vi "Switch Scalar Type.vi"(8 "error in (no error)":errorcluster, 11 "Node Ptr":u64 format="%.0x") -> (0 "error out":errorcluster)   [LabVIEW 2016, in "FPGA Addon System Explorer.lvlib"]
uses:
  FPGA Addon System Explorer.lvlib
  <vilib>/NI Veristand/Custom Device API/Custom Device Channel.ctl
  <vilib>/NI Veristand/Custom Device API/Custom Device Channel Type.ctl
  Shared/Constants.vi
  <vilib>/NI Veristand/Custom Device API/Get Item Property (String).vi
  <vilib>/NI Veristand/Custom Device API/Set Item Property (String).vi
  <vilib>/NI VeriStand/Custom Device API/Custom Device API.lvlib
  Shared/FPGA Addon Shared.lvlib
  <vilib>/NI VeriStand/Custom Device Tools/Custom Device Utility Library/Custom Device Utility Library.lvlib
panel:
  in  "Tag":string
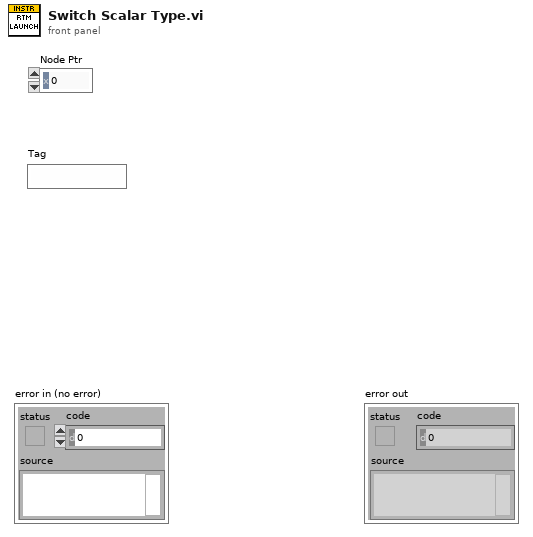
[diagram p1: front panel]
types:
  T1 = typedef "Custom Device API.lvlib/Custom Device Item Ref.ctl" = u64
  T2 = typedef "Custom Device API.lvlib/Custom Device Item Info.ctl" = cluster{"Name":string, "Is Channel":bool, "GUID":string, "Is Waveform":bool}
  T3 = typedef "Custom Device API.lvlib/Custom Device Channel.ctl" = cluster{"Type":T4, "Units":string, "Default Value":dbl, "Faultable":bool, "Scalable":bool}
  T4 = typedef "Custom Device API.lvlib/Custom Device Channel Type.ctl" = enum16{"Input", "Output"}
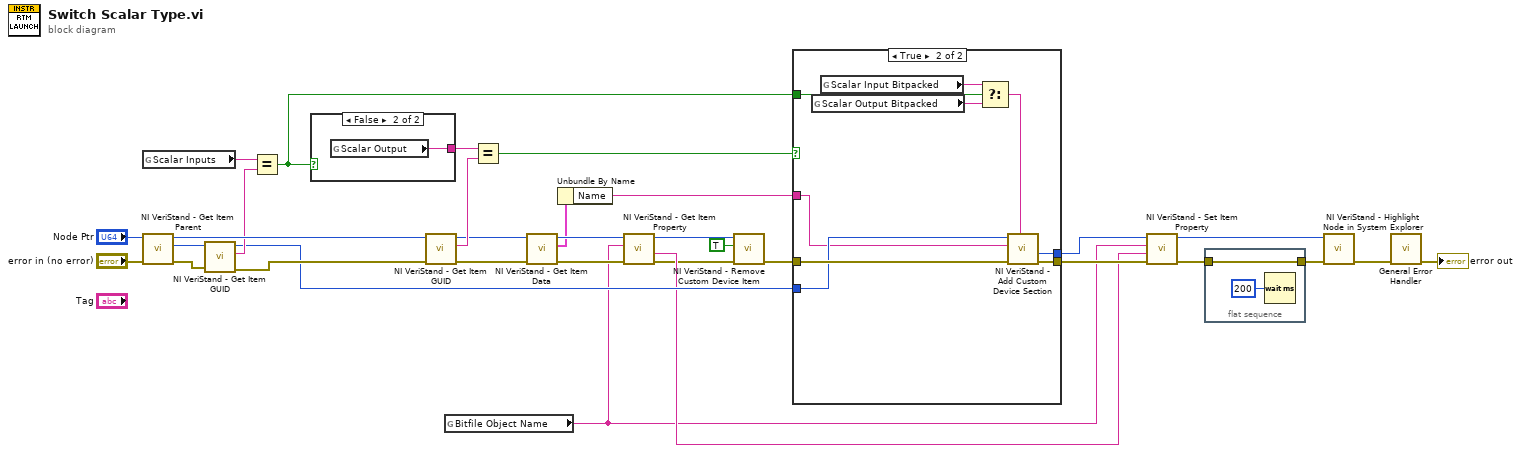
[diagram p0: block diagram]
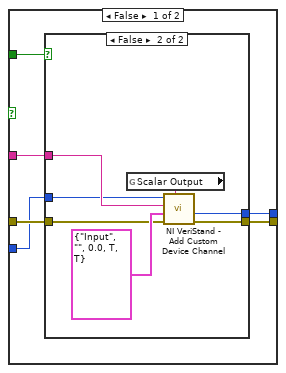
[diagram p2: hidden frame]
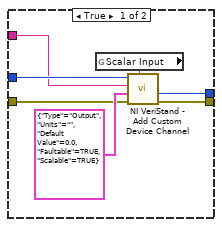
[diagram p3: hidden frame]
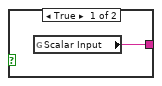
[diagram p4: hidden frame]
diagram:
  n1 = global read "Constants.vi" "Scalar Inputs"() -> (w23:string)
  n2 = call <vilib>:"NI VeriStand - Get Item Parent.vi"("error in (no error)"="error in (no error)", "Item Ref in"="Node Ptr") -> ("error out"=w25:errorcluster, "Parent Ref"=w26:T1, "Item Ref out"=w28:T1)  [unwired: 6 in, 1 out]
  n3 = call <vilib>:"NI VeriStand - Get Item GUID.vi"("error in (no error)"=w25, "Item Ref in"=w26) -> ("error out"=w22:errorcluster, "GUID"=w24:string, "Item Ref out"=w19:T1)  [unwired: 7 in]
  n4 = Equal?(x=w23, y=w24) -> (x = y?=w17:bool)
  n5 = case shown="False" w17 {
    tunnel: [w33 w34] -> w29
    frame True {
      n6 = global read "Constants.vi" "Scalar Input"() -> (w33:string)
    }
    frame False {
      n7 = global read "Constants.vi" "Scalar Output"() -> (w34:string)
    }
  }
  n8 = call <vilib>:"NI VeriStand - Get Item GUID.vi"("error in (no error)"=w22, "Item Ref in"=w28) -> ("error out"=w9:errorcluster, "GUID"=w32:string, "Item Ref out"=w11:T1)  [unwired: 7 in]
  n9 = global read "Constants.vi" "Bitfile Object Name"() -> (w5:string)
  n10 = Equal?(x=w29, y=w32) -> (x = y?=w18:bool)
  n11 = call <vilib>:"NI VeriStand - Get Item Data.vi"("error in (no error)"=w9, "Item Ref in"=w11) -> ("error out"=w8:errorcluster, "Item Info"=w7:T2, "Item Ref out"=w10:T1)  [unwired: 6 in, 1 out]
  n12 = Unbundle By Name(w7) -> ("Name"=w6:string)
  n13 = call-poly <vilib>:"NI VeriStand - Get Item Property.vi"("error in (no error)"=w8, "Property Name"=w5, "Item Ref in"=w10) -> ("error out"=w13:errorcluster, "Value"=w14:string, "Item Ref out"=w12:T1)  [unwired: 5 in, 1 out]
  n14 = call <vilib>:"NI VeriStand - Remove Custom Device Item.vi"("error in (no error)"=w13, "Force Delete (F)"=TRUE, "Item Ref in"=w12) -> ("error out"=w20:errorcluster)  [unwired: 7 in, 1 out]
  n15 = case shown="True" w18 {
    tunnel: w20 -> [w40 w63]
    tunnel: w19 -> [w36 w62]
    tunnel: w17 -> [w37 w60]
    tunnel: [w39 w58] -> w16
    tunnel: [w38 w57] -> w15
    tunnel: w6 -> [w35 w56]
    frame False {
      n16 = case shown="False" w37 {
        tunnel: w40 -> [w45 w52]
        tunnel: [w44 w51] -> w39
        tunnel: [w43 w50] -> w38
        tunnel: w36 -> [w42 w48]
        tunnel: w35 -> [w41 w49]
        frame True {
          n17 = global read "Constants.vi" "Scalar Input"() -> (w47:string)
          n18 = call <vilib>:"NI VeriStand - Add Custom Device Channel.vi"("GUID (Default Channel)"=w47, "error in (no error)"=w45, "Channel"=T3 {"Type"=enum."Output", "Units"="", "Default Value"=0.0, "Faultable"=TRUE, "Scalable"=TRUE}, "Channel Name"=w41, "Parent Ref in"=w42) -> ("error out"=w44:errorcluster, "Channel Ref"=w43:T1)  [unwired: 3 in, 2 out]
        }
        frame False {
          n19 = global read "Constants.vi" "Scalar Output"() -> (w54:string)
          n20 = call <vilib>:"NI VeriStand - Add Custom Device Channel.vi"("GUID (Default Channel)"=w54, "error in (no error)"=w52, "Channel"=T3 {"Type"=enum."Input", "Units"="", "Default Value"=0.0, "Faultable"=TRUE, "Scalable"=TRUE}, "Channel Name"=w49, "Parent Ref in"=w48) -> ("error out"=w51:errorcluster, "Channel Ref"=w50:T1)  [unwired: 3 in, 2 out]
        }
      }
    }
    frame True {
      n21 = global read "Constants.vi" "Scalar Output Bitpacked"() -> (w59:string)
      n22 = global read "Constants.vi" "Scalar Input Bitpacked"() -> (w61:string)
      n23 = Select(t=w61, s=w60, f=w59) -> (s? t:f=w55:string)
      n24 = call <vilib>:"NI VeriStand - Add Custom Device Section.vi"("GUID (Default Section)"=w55, "error in (no error)"=w63, "Section Name"=w56, "Parent Ref in"=w62) -> ("error out"=w58:errorcluster, "Section Ptr"=w57:T1)  [unwired: 4 in, 2 out]
    }
  }
  n25 = call-poly <vilib>:"NI VeriStand - Set Item Property.vi"("error in (no error)"=w16, "Value"=w14, "Property Name"=w5, "Item Ref in"=w15) -> ("error out"=w1:errorcluster, "Item Ref out"=w3:T1)  [unwired: 5 in, 1 out]
  n26 = flat-sequence {
    tunnel: [w65] -> w2
    tunnel: w1 -> [w65]
    frame #0 {
      n27 = Wait (ms)(milliseconds to wait=u32 200) -> ()  [unwired: 1 out]
    }
  }
  n28 = call <vilib>:"NI VeriStand - Highlight Node in System Explorer.vi"("error in (no error)"=w2, "Item Ref in"=w3) -> ("error out"=w4:errorcluster)  [unwired: 8 in, 1 out]
  n29 = call <vilib>:"General Error Handler.vi"("error in (no error)"=w4) -> ("error out"=→"error out":errorcluster)  [unwired: 10 in, 4 out]
